vi "ExOpenCamTestGlobal.vi"() -> ()   [LabVIEW 2010]
uses:
  GlbCamHndls.vi
panel:
  out "Array":bool[](array[boolean])
  out "Total camera array size":u32
  out "error out":errorcluster
  in  "error in (no error)":errorcluster
  in  "Camera Number to open":u32=1 min=1 step=1
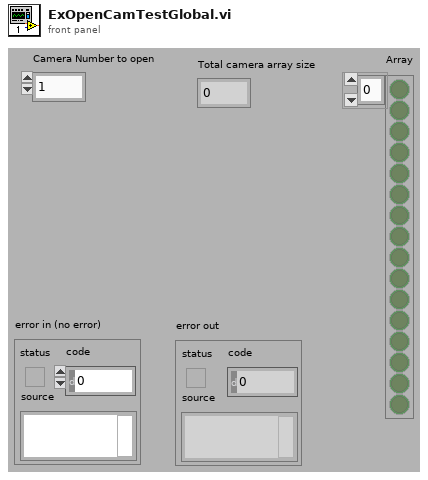
[diagram p1: front panel]
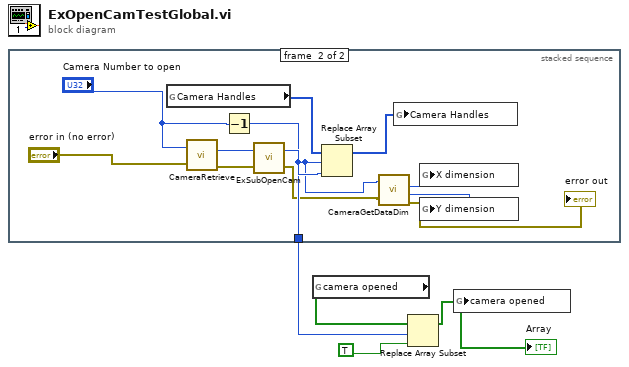
[diagram p0: block diagram]
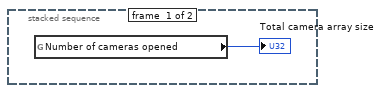
[diagram p2: hidden frame]
diagram:
  n1 = stacked-sequence {
    tunnel: [_ w8] -> w4
    frame #0 {
      n2 = global read "GlbCamHndls.vi" "Number of cameras opened"() -> (→"Total camera array size":u32)
    }
    frame #1 {
      n3 = global read "GlbCamHndls.vi" "Camera Handles"() -> (w14:u32[])
      n4 = call <userlib>:"CameraRetrieve.vi"("error in"="error in (no error)", "Camera Index"="Camera Number to open") -> ("error out"=w16:errorcluster, "Device ID"=w15:u32)
      n5 = Decrement(x="Camera Number to open") -> (x-1=w8:u32)
      n6 = call "ExSubOpenCam.vi"("error in (no error)"=w16, "Camera Device ID"=w15) -> ("error out"=w7:errorcluster, "Camera Handle"=w13:u32)
      n7 = Replace Array Subset(array=w14, new element=w13, index=w8) -> (w11:u32[])
      n8 = call <userlib>:"CameraGetDataDim.vi"("Camera Handle"=w8, "error in"=w7) -> ("Xdim"=w9:u32, "Ydim"=w10:u32, "error out"=→"error out":errorcluster)  [unwired: 1 out]
      n9 = global write "GlbCamHndls.vi" "Camera Handles"(w11) -> ()
      n10 = global write "GlbCamHndls.vi" "X dimension"(w9) -> ()
      n11 = global write "GlbCamHndls.vi" "Y dimension"(w10) -> ()
    }
  }
  n12 = global read "GlbCamHndls.vi" "camera opened"() -> (w2:bool[])
  n13 = Replace Array Subset(array=w2, new element=TRUE, index=w4) -> (w1:bool[])
  "Array" <- w1
  n14 = global write "GlbCamHndls.vi" "camera opened"(w1) -> ()
